vi "stop.vi"(0 "Boolean":bool) -> ()   [LabVIEW 2013]
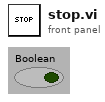
[diagram p1: front panel]
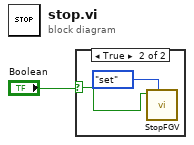
[diagram p0: block diagram]
diagram:
  n1 = case shown="True" "Boolean" {
    selector: "Boolean" -> [_ w2]
    frame False {
    }
    frame True {
      n2 = call "StopFGV.vi"("Command"=enum16{"set", "get", "init"}."set", "Stop"=w2) -> ()  [unwired: 8 in, 2 out]
    }
  }
